vi "_GetLVInfo.vi"(8 "error in (no error)":errorcluster, 10 "32bit(T)/64bit(F)":bool, 11 "Array":path[](array[path])) -> (0 "error out":errorcluster, 3 "LabVIEW Info":T1[](array[typedef]))   [LabVIEW 2014, in "application.lvclass"]
uses:
  application.lvclass
  control/DEF-LabVIEW INFO.ctl
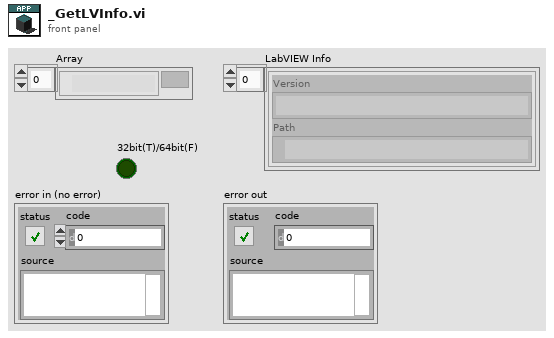
[diagram p1: front panel]
types:
  T1 = typedef "application.lvclass/DEF-LabVIEW INFO.ctl" = cluster{"Version":string, "Path":path}
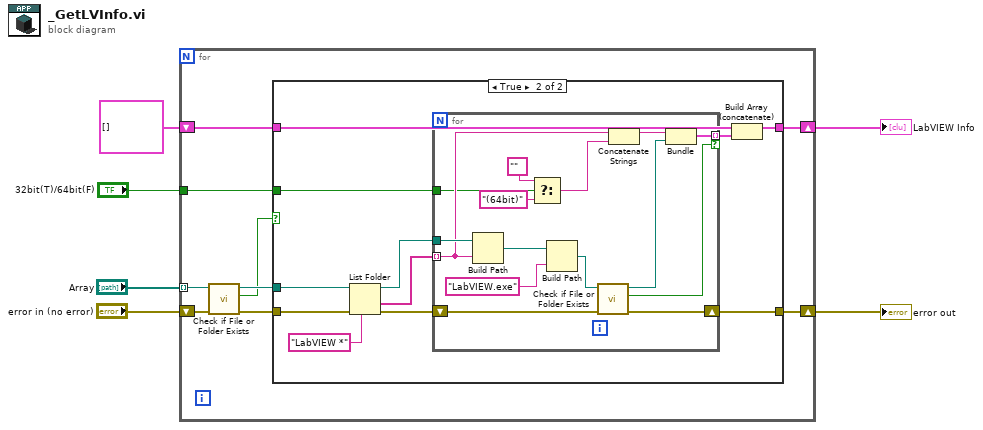
[diagram p0: block diagram]
diagram:
  n1 = for {
    tunnel: "Array" -> [w15] mode=indexing
    shift-right: [w11] -> w4
    shift-left: T1[] [] ("LabVIEW Info") -> [w10]
    shift-right: [w9] -> w3
    shift-left: "error in (no error)" -> [w8]
    tunnel: "32bit(T)/64bit(F)" -> [w7]
    n2 = call <vilib>:"Check if File or Folder Exists.vi"("error in (no error)"=w8, "path"=w15) -> ("error out"=w13:errorcluster, "file or folder exists?"=w12:bool, "dup path"=w14:path)  [unwired: 7 in]
    n3 = case shown="True" w12 {
      tunnel: w14 -> [_ w21]
      tunnel: w13 -> [w16 w28]
      tunnel: [w17 w25] -> w11
      tunnel: w10 -> [w17 w24]
      tunnel: [w16 w23] -> w9
      tunnel: w7 -> [_ w18]
      frame False {
      }
      frame True {
        n4 = List Folder(path=w21, pattern="LabVIEW *", error in=w28) -> (path out=w20:path, folder names=w19:string[], error out=w27:errorcluster)  [unwired: 1 in, 1 out]
        n5 = for {
          tunnel: w20 -> [w43]
          tunnel: w19 -> [w38] mode=indexing
          tunnel: [w36] -> w26 mode=indexing if=w37
          shift-right: [w34] -> w23
          shift-left: w27 -> [w42]
          tunnel: w18 -> [w33]
          n6 = Build Path(base path=w43, name or relative path=w38) -> (appended path=w41:path)
          n7 = Select(t="", s=w33, f="(64bit)") -> (s? t:f=w29:string)
          n8 = Build Path(base path=w41, name or relative path="LabVIEW.exe") -> (appended path=w39:path)
          n9 = call <vilib>:"Check if File or Folder Exists.vi"("error in (no error)"=w42, "path"=w39) -> ("error out"=w34:errorcluster, "file or folder exists?"=w37:bool, "dup path"=w35:path)  [unwired: 7 in]
          n10 = Concatenate Strings(w38, w29) -> (w30:string)
          n11 = Bundle(w30, "dup path"=w35) -> (w36:cluster{string, "dup path":path})  [unwired: 1 in]
        }
        n12 = Build Array (concatenate)(w24, w26) -> (w25:T1[])
      }
    }
  }
  "LabVIEW Info" <- w4
  "error out" <- w3
